vi "Intake Outtake.vi"(7 "Description":string, 8 "Command Info In":T1, 11 "Setpoint":dbl) -> (0 "Command Info Out":T1)   [LabVIEW 2019]
doc: "This template is useful for immediate subsystem actions that do not need deadband filtering\n\nBe sure to right-click and select New from Template and save with a new command name."
uses:
  <vilib>/Rock Robotics/WPI/Framework/Command Status Info.ctl
  <vilib>/Rock Robotics/WPI/Framework/Completion Status.ctl
  <vilib>/Rock Robotics/WPI/Framework/Completion Notifier.ctl
  Implementation/Intake Setpoints.ctl
  Implementation/Intake Operations.ctl
  Intake Support Code/Pivot Position.ctl
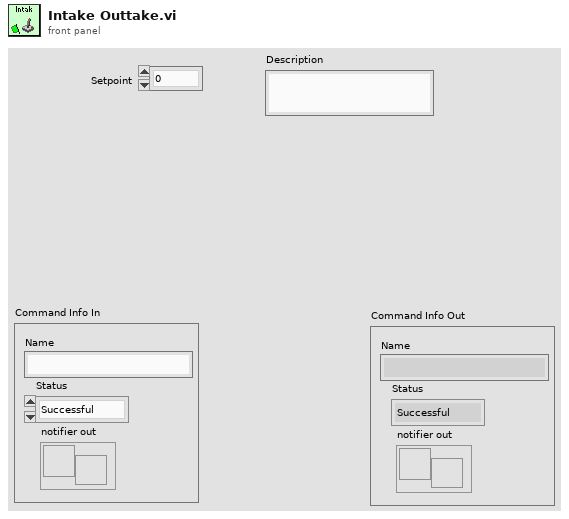
[diagram p1: front panel]
types:
  T1 = typedef "Command Status Info.ctl" = cluster{"Name":string, "Status":T2, "notifier out":T3}
  T2 = typedef "Completion Status.ctl" = enum16{"Successful", "Aborted", "Incomplete"}
  T3 = typedef "Completion Notifier.ctl" = refnum<notifier>
  T4 = typedef "Intake Setpoints.ctl" = cluster{"Operation":T5, "Setpoint":dbl, "Pivot Position":T6}
  T5 = typedef "Intake Operations.ctl" = enum16{"Reserve", "Read Current", "Immediate", "Spin Rollers", "Pivot Position", "Intake Forever"}
  T6 = typedef "Pivot Position.ctl" = enum16{"Down", "Up"}
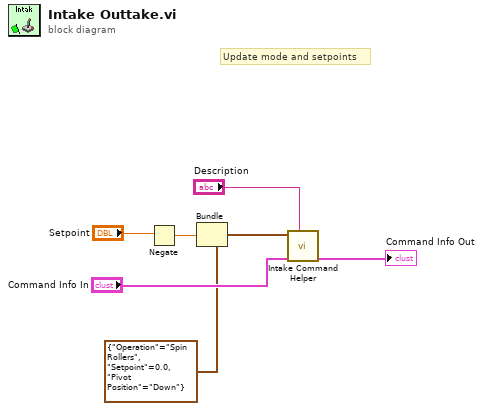
[diagram p0: block diagram]
diagram:
  # "Update mode and setpoints"
  n1 = Negate(x="Setpoint") -> (-x=w1:dbl)
  n2 = Bundle(cluster=T4 {"Operation"=enum."Spin Rollers", "Setpoint"=0.0, "Pivot Position"=enum."Down"} ("SubSystem Data"), "Setpoint"=w1) -> (w3:T4)  [unwired: 2 in]
  n3 = call "Intake Command Helper.vi"("Description"="Description", "Command Info In"="Command Info In", "SubSystem Data"=w3) -> ("Command Info Out"=→"Command Info Out":T1)  [unwired: 6 in, 2 out]
